vi "testTelToClient.vi"(8 "error in (no error)":errorcluster) -> (0 "error out":errorcluster)   [LabVIEW 2018]
doc: "Test the telToClient.vi"
uses:
  src/TcpServer/TcpServer.lvclass
  src/TcpServerTel/typedef/queueOptionsTypeDef.ctl
  src/TcpServerTel/typedef/enqueueOptionsTypeDef.ctl
  src/TcpServerTel/typedef/telTypeDef.ctl
  src/TcpServer/TcpServer.lvclass/TcpServer.ctl
  src/TcpServerBase/TcpServerBase.lvclass/TcpServerBase.ctl
  src/TcpServerTel/TcpServerTel.lvclass
  home/pcortes/github/ts_labview_tcp_json/src/TcpServerBase/TcpServerBase.lvclass
  <vilib>/addons/_JKI Toolkits/Caraya/classes/Assert/Assert Equal Type_Variant.vi
  <vilib>/addons/_JKI Toolkits/Caraya/classes/Test/Test.lvclass
  <vilib>/addons/_JKI Toolkits/Caraya/classes/Assert/Assert.lvclass
  src/TcpServerBase/TcpServerBase.lvclass
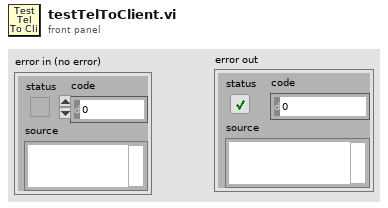
[diagram p1: front panel]
types:
  T1 = typedef "TcpServerTel.lvclass/telTypeDef.ctl" = cluster{"name":string, "telDetails":string}
  T2 = typedef "TcpServerTel.lvclass/queueOptionsTypeDef.ctl" = cluster{"EnqueueOptions":T3, "Timeout (ms)":i32}
  T3 = typedef "TcpServerTel.lvclass/enqueueOptionsTypeDef.ctl" = enum16{"lossy enqueue", "normal enqueue"}
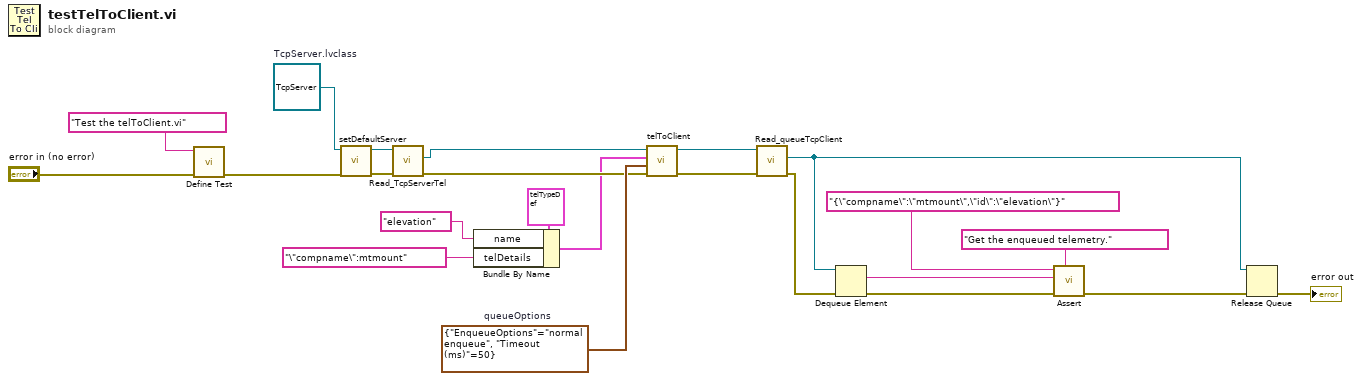
[diagram p0: block diagram]
diagram:
  w16 = T2 {"EnqueueOptions"=enum."normal enqueue", "Timeout (ms)"=50}  # queueOptions
  w14 = refnum<class "TcpServer.lvclass"> refnum  # TcpServer.lvclass
  n1 = call <vilib>:"Define Test.vi"("error in (no error)"="error in (no error)", "Label (VI Title)"="Test the telToClient.vi") -> ("error out"=w15:errorcluster)  [unwired: 9 in]
  n2 = call "setDefaultServer.vi"("error in (no error)"=w15, "TcpServer.lvclass"=w14) -> ("error out"=w13:errorcluster, "tcpServer out"=w11:refnum<class "TcpServer.lvclass">)  [unwired: 8 in]
  n3 = call "Read_TcpServerTel.vi"("error in (no error)"=w13, "TcpServer in"=w11) -> ("error out"=w12:errorcluster, "TcpServerTel.lvclass"=w9:refnum<class "TcpServerTel.lvclass">)  [unwired: 7 in, 1 out]
  n4 = Bundle By Name(cluster=T1 {"name"="elevation", "telDetails"="\"compName\":\"MTMount\""} ("Telemetry"), "name"="elevation", "telDetails"="\"compname\":mtmount") -> (w6:T1)
  n5 = call "telToClient.vi"("error in (no error)"=w12, "queueOptions"=w16, "Telemetry"=w6, "TcpServerTel in"=w9) -> ("error out"=w4:errorcluster, "TcpServerTel out"=w5:refnum<class "TcpServerTel.lvclass">)  [unwired: 6 in]
  n6 = call "Read_queueTcpClient.vi"("error in (no error)"=w4, "TcpServerBase in"=w5) -> ("error out"=w3:errorcluster, "tcpClientQueue"=w2:refnum<queue>)  [unwired: 7 in, 1 out]
  n7 = Dequeue Element(queue=w2, error in (no error)=w3) -> (element=w18:string, error out=w17:errorcluster)  [unwired: 1 in, 2 out]
  n8 = call-poly <vilib>:"Assert.vi"("Label"="Get the enqueued telemetry.", "error in (no error)"=w17, "Y"=w18, "X"="{\"compname\":\"mtmount\",\"id\":\"elevation\"}" ("telDetails")) -> ("error out"=w21:errorcluster)  [unwired: 7 in]
  n9 = Release Queue(queue=w2, error in (no error)=w21) -> (error out=→"error out":errorcluster)  [unwired: 1 in, 2 out]
